vi "Body.vi"() -> ()   [LabVIEW 2011]
uses:
  <vilib>/Utility/miscctls.llb/LVPointTypeDef.ctl
  Globals/Global VI.vi
panel:
  out "Access Levels":i32[](array[numeric])
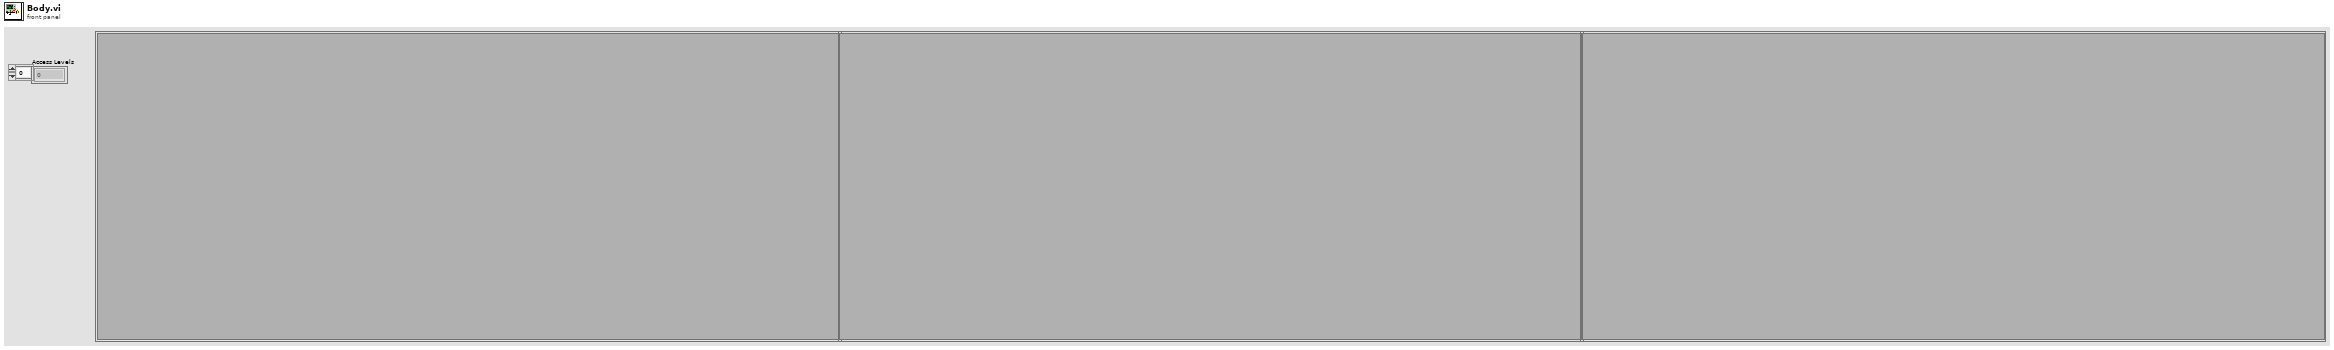
[diagram p1: front panel]
types:
  T1 = typedef "LVPointTypeDef.ctl" = cluster{"Horizontal":i16, "Vertical":i16}
  T2 = enum32{"Bad", "Idle", "Run top level", "Running"}
  T3 = enum8{"Enabled", "Disabled", "Disabled and Grayed Out"}
  T4 = enum16{"Always On", "Always Off", "Off While Running"}
  T5 = typedef "LVAllMonitorsDisplayTypeDef.ctl" = cluster{"Bounds":cluster{"Left":i16, "Top":i16, "Right":i16, "Bottom":i16}, "Depth":i16}[]
  T6 = typedef "LVRectTypeDef.ctl" = cluster{"left":i16, "top":i16, "right":i16, "bottom":i16}
  T7 = cluster{"Bounds":cluster{"Left":i16, "Top":i16, "Right":i16, "Bottom":i16}, "Depth":i16}
  T8 = typedef "LVBoundsTypeDef.ctl" = cluster{"Width":u32, "Height":u32}
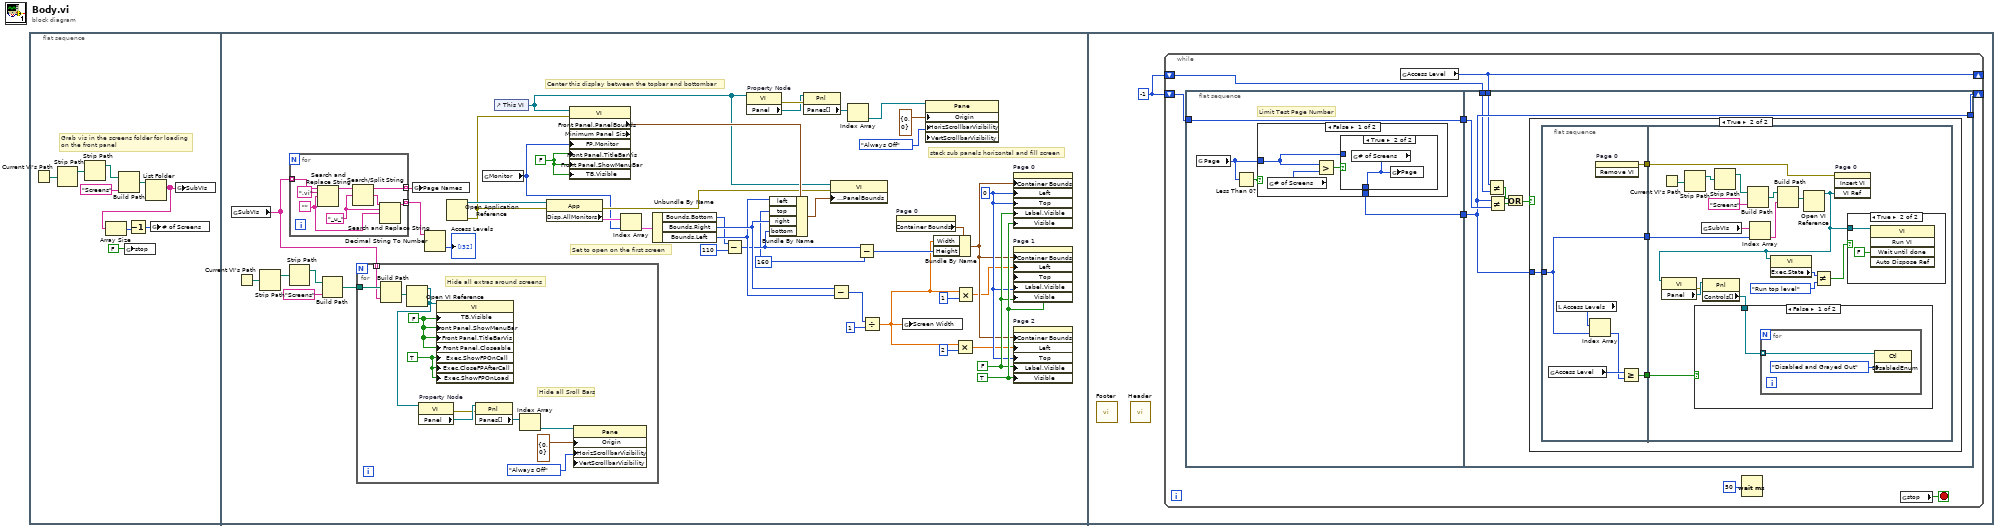
[diagram p0: block diagram]
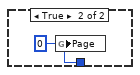
[diagram p3: hidden frame]
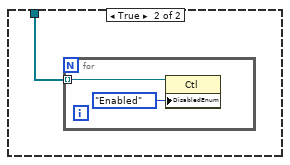
[diagram p6: hidden frame]
diagram:
  n1 = flat-sequence {
    frame #0 {
      # "Grab vis in the screens folder for loading\non the front panel"
      n2 = Current VI's Path() -> (path=w8:path)
      n3 = Strip Path(path=w8) -> (stripped path=w6:path)  [unwired: 1 out]
      n4 = Strip Path(path=w6) -> (stripped path=w5:path)  [unwired: 1 out]
      n5 = Build Path(base path=w5, name or relative path="Screens") -> (appended path=w7:path)
      n6 = global write "Global VI.vi" "stop"(FALSE ("stop")) -> ()
      n7 = List Folder(path=w7) -> (filenames=w2:string[])  [unwired: 3 in, 3 out]
      n8 = Array Size(array=w2) -> (size(s)=w3:i32)
      n9 = Decrement(x=w3) -> (x-1=w4:i32)
      n10 = global write "Global VI.vi" "# of Screens"(w4) -> ()
      n11 = global write "Global VI.vi" "SubVIs"(w2) -> ()
    }
    frame #1 {
      w13 = T4."Always Off" ("Horizontal Scrollbar Visibility")
      w15 = FALSE ("Front Panel Window:Title Bar Visible")
      w46 = TRUE ("Label.Visible")
      w45 = FALSE ("Label.Visible")
      w44 = 0 ("Position:Left")
      w36 = i16 160 ("top")
      # "Set to open on the first screen"
      # "stack sub panels horizontal and fill screen"
      # "Center this display between the topbar and bottombar"
      n12 = global read "Global VI.vi" "SubVIs"() -> (w21:string[])
      n13 = Current VI's Path() -> (path=w51:path)
      n14 = Strip Path(path=w51) -> (stripped path=w18:path)  [unwired: 1 out]
      n15 = for {
        tunnel: w21 -> [w73] mode=indexing
        tunnel: [w70] -> w12 mode=indexing
        tunnel: [w66] -> w11 mode=indexing
        w68 = "_u_" ("search string/char (-)")
        w67 = ""
        n16 = Search and Replace String(input string=w73, search string=".vi", replace string=w67) -> (result string=w71:string)  [unwired: 5 in, 3 out]
        n17 = Search/Split String(string=w71, search string/char (-)=w68) -> (substring before match=w70:string, match + rest of string=w69:string)  [unwired: 1 in, 1 out]
        n18 = Search and Replace String(input string=w69, search string=w68, replace string=w67) -> (result string=w66:string)  [unwired: 5 in, 3 out]
      }
      n19 = Strip Path(path=w18) -> (stripped path=w17:path)  [unwired: 1 out]
      n20 = Build Path(base path=w17, name or relative path="Screens") -> (appended path=w53:path)
      n21 = for {
        tunnel: w53 -> [w64]
        tunnel: w21 -> [w63] mode=indexing
        w60 = T4."Always Off" ("Horizontal Scrollbar Visibility")
        w61 = TRUE ("Execution:Show Front Panel On Call")
        w62 = FALSE ("Tool Bar:Visible")
        # "Hide all extras around screens"
        # "Hide all Sroll Bars"
        n22 = Build Path(base path=w64, name or relative path=w63) -> (appended path=w65:path)
        n23 = Open VI Reference(vi path=w65) -> (vi reference=w54:refnum<vi>)  [unwired: 5 in, 1 out]
        n24 = property on="Property Node" class="VI"(reference=w54) -> (error out=w57:errorcluster, "Panel"=w58:refnum<vi>)  [unwired: 1 in, 1 out]
        n25 = property class="VI"(reference=w54, "TB.Visible"=w62, "Front Panel.ShowMenuBar"=w62, "Front Panel.TitleBarVis"=w62, "Front Panel.Closeable"=w62, "Exec.ShowFPOnCall"=w61, "Exec.CloseFPAfterCall"=w61, "Exec.ShowFPOnLoad"=w61) -> ()  [unwired: 1 in, 2 out]
        n26 = property class="Pnl"(reference=w58, error in=w57) -> ("Panes[]"=w59:refnum<vi>[])  [unwired: 2 out]
        n27 = Index Array "Index Array"(array=w59) -> (element=w55:refnum<vi>)  [unwired: 1 in]
        n28 = property class="Pane"(reference=w55, "Origin"=T1 {"Horizontal"=0, "Vertical"=0}, "HorizScrollbarVisibility"=w60, "VertScrollbarVisibility"=w60) -> ()  [unwired: 1 in, 2 out]
      }
      n29 = global write "Global VI.vi" "Page Names"(w12) -> ()
      n30 = Decimal String To Number(string=w11) -> (number=→"Access Levels":i32[])  [unwired: 2 in, 1 out]
      n31 = Open Application Reference() -> (0:w27:errorcluster, 3:w33:refnum<vi>)  [unwired: 4 in]
      n32 = global read "Global VI.vi" "Monitor"() -> (w20:u16)
      n33 = control-ref of="This VI"() -> (w16:refnum<vi>)
      n34 = property class="App"(reference=w33, error in=w27) -> (error out=w24:errorcluster, "Disp.AllMonitors"=w23:T5)  [unwired: 1 out]
      n35 = property class="VI" props=["Front Panel.PanelBounds", "Minimum Panel Size", "FP.Monitor", "Front Panel.TitleBarVis", "Front Panel.ShowMenuBar", "TB.Visible"](reference=w16, error in=w27, "FP.Monitor"=w20, "Front Panel.TitleBarVis"=w15, "Front Panel.ShowMenuBar"=w15, "TB.Visible"=w15) -> ("Front Panel.PanelBounds"=w26:T6)  [unwired: 3 out]
      n36 = Index Array(array=w23, index=w20) -> (element=w22:T7)
      n37 = Unbundle By Name(w22) -> ("Bounds.Bottom"=w28:i16, "Bounds.Right"=w48:i16, "Bounds.Left"=w47:i16)
      n38 = Subtract(x=w28, y=i16 110) -> (x-y=w37:i16)
      n39 = property on="Property Node" class="VI"(reference=w16) -> (error out=w31:errorcluster, "Panel"=w30:refnum<vi>)  [unwired: 1 in, 1 out]
      n40 = Bundle By Name(cluster=w26, "left"=w47, "top"=w36, "right"=w48, "bottom"=w37) -> (w25:T6)
      n41 = property class="Pnl"(reference=w30, error in=w31) -> ("Panes[]"=w14:refnum<vi>[])  [unwired: 2 out]
      n42 = property class="VI"(reference=w16, error in=w24, "Front Panel.PanelBounds"=w25) -> ()  [unwired: 2 out]
      n43 = Subtract(x=w48, y=w47) -> (x-y=w49:i16)
      n44 = Index Array "Index Array"(array=w14) -> (element=w34:refnum<vi>)  [unwired: 1 in]
      n45 = Subtract(x=w37, y=w36) -> (x-y=w38:i16)
      n46 = Divide(x=w49, y=i16 1) -> (x/y=w19:dbl)
      n47 = property on="Page 0" class="SubPnl"() -> ("Container Bounds"=w35:T8)  [unwired: 2 in, 2 out]
      n48 = global write "Global VI.vi" "Screen Width"(w19) -> ()
      n49 = property class="Pane"(reference=w34, "Origin"=T1 {"Horizontal"=0, "Vertical"=0}, "HorizScrollbarVisibility"=w13, "VertScrollbarVisibility"=w13) -> ()  [unwired: 1 in, 2 out]
      n50 = Bundle By Name(cluster=w35, "Width"=w19, "Height"=w38) -> (w41:T8)
      n51 = Multiply(x=w19, y=i16 2) -> (x*y=w43:dbl)
      n52 = Multiply(x=w19, y=i16 1) -> (x*y=w40:dbl)
      n53 = property on="Page 0" class="SubPnl"("Container Bounds"=w41, "Left"=w44, "Top"=w44, "Label.Visible"=w45, "Visible"=w46) -> ()  [unwired: 2 in, 2 out]
      n54 = property on="Page 1" class="SubPnl"("Container Bounds"=w41, "Left"=w40, "Top"=w44, "Label.Visible"=w45, "Visible"=w46) -> ()  [unwired: 2 in, 2 out]
      n55 = property on="Page 2" class="SubPnl"("Container Bounds"=w41, "Left"=w43, "Top"=w44, "Label.Visible"=w45, "Visible"=w46) -> ()  [unwired: 2 in, 2 out]
    }
    frame #2 {
      w74 = i16 -1 ("Page")
      n56 = call "Footer.vi"() -> ()  [unwired: 12 in]
      n57 = call "Header.vi"() -> ()  [unwired: 12 in]
      n58 = while {
        shift-right: [w79] -> _
        shift-left: w74 -> [w80]
        shift-right: [w77] -> _
        shift-left: w74 -> [w76]
        stop <- w82 stop-if-true
        n59 = flat-sequence {
          tunnel: [w85] -> w81
          tunnel: w80 -> [w85]
          tunnel: [w83] -> w78
          tunnel: w81 -> [w100]
          tunnel: [w99] -> w79
          tunnel: w78 -> [w99]
          tunnel: w77 -> [w98]
          tunnel: w76 -> [w97]
          frame #0 {
            # "Limit Test Page Number"
            n60 = global read "Global VI.vi" "Page"() -> (w84:i16)
            n61 = Less Than 0?(x=w84) -> (x < 0?=w86:bool)
            n62 = case shown="False" w86 {
              tunnel: w84 -> [w87 _]
              tunnel: [w88 w93] -> w83
              frame False {
                n63 = global read "Global VI.vi" "# of Screens"() -> (w89:i16)
                n64 = Greater?(x=w87, y=w89) -> (0:w90:bool)
                n65 = case shown="True" w90 {
                  tunnel: [w91 w92] -> w88
                  tunnel: w87 -> [w91 _]
                  frame False {
                  }
                  frame True {
                    n66 = global read "Global VI.vi" "# of Screens"() -> (w92:i16)
                    n67 = global write "Global VI.vi" "Page"(w92) -> ()
                  }
                }
              }
              frame True {
                w93 = i16 0 ("Page")
                n68 = global write "Global VI.vi" "Page"(w93) -> ()
              }
            }
          }
          frame #1 {
            n69 = Not Equal?(x=w98, y=w97) -> (x != y?=w94:bool)
            n70 = Not Equal?(x=w99, y=w100) -> (x != y?=w95:bool)
            n71 = Or(x=w94, y=w95) -> (x .or. y?=w96:bool)
            n72 = case shown="True" w96 {
              tunnel: w99 -> [_ w103]
              frame False {
              }
              frame True {
                n73 = flat-sequence {
                  tunnel: [w110] -> w104
                  tunnel: w103 -> [w106]
                  tunnel: [w106] -> w102
                  tunnel: [w108] -> w101
                  tunnel: w104 -> [w120]
                  tunnel: w102 -> [w119]
                  tunnel: w101 -> [w115]
                  frame #0 {
                    n74 = global read "Global VI.vi" "Access Level"() -> (w109:u16)
                    n75 = local read "Access Levels"() -> (w107:i32[])
                    n76 = Index Array(array=w107, index=w106) -> (element=w105:i32)
                    n77 = invoke on="Page 0" class="SubPnl" method="Remove VI"() -> (error out=w110:errorcluster)  [unwired: 3 in, 2 out]
                    n78 = Greater Or Equal?(x=w109, y=w105) -> (x >= y?=w108:bool)
                  }
                  frame #1 {
                    n79 = Current VI's Path() -> (path=w127:path)
                    n80 = Strip Path(path=w127) -> (stripped path=w126:path)  [unwired: 1 out]
                    n81 = global read "Global VI.vi" "SubVIs"() -> (w122:string[])
                    n82 = Strip Path(path=w126) -> (stripped path=w125:path)  [unwired: 1 out]
                    n83 = Build Path(base path=w125, name or relative path="Screens") -> (appended path=w123:path)
                    n84 = Index Array(array=w122, index=w119) -> (element=w121:string)
                    n85 = Build Path(base path=w123, name or relative path=w121) -> (appended path=w124:path)
                    n86 = Open VI Reference(vi path=w124) -> (vi reference=w114:refnum<vi>)  [unwired: 5 in, 1 out]
                    n87 = property class="VI"(reference=w114) -> (error out=w117:errorcluster, "Panel"=w118:refnum<vi>)  [unwired: 1 in, 1 out]
                    n88 = property class="Pnl"(reference=w118, error in=w117) -> ("Controls[]"=w116:refnum<vi>[])  [unwired: 2 out]
                    n89 = case shown="False" w115 {
                      tunnel: w116 -> [w131 w134]
                      frame False {
                        n90 = for {
                          tunnel: w131 -> [w133] mode=indexing
                          n91 = property class="Ctl"(reference=w133, "DisabledEnum"=T3."Disabled and Grayed Out" ("Disabled")) -> ()  [unwired: 1 in, 2 out]
                        }
                      }
                      frame True {
                        n92 = for {
                          tunnel: w134 -> [w136] mode=indexing
                          n93 = property class="Ctl"(reference=w136, "DisabledEnum"=T3."Enabled" ("Disabled")) -> ()  [unwired: 1 in, 2 out]
                        }
                      }
                    }
                    n94 = property class="VI"(reference=w114) -> ("Exec.State"=w112:T2)  [unwired: 1 in, 2 out]
                    n95 = Not Equal?(x=w112, y=T2."Run top level" ("Execution:State")) -> (x != y?=w111:bool)
                    n96 = invoke on="Page 0" class="SubPnl" method="Insert VI"(error in=w120, "VI Ref"=w114) -> ()  [unwired: 2 in, 4 out]
                    n97 = case shown="True" w111 {
                      tunnel: w114 -> [_ w130]
                      frame False {
                      }
                      frame True {
                        n98 = invoke class="VI" method="Run VI"(reference=w130, "Wait until done"=FALSE ("Wait Until Done")) -> ()  [unwired: 3 in, 5 out]
                      }
                    }
                  }
                }
              }
            }
          }
        }
        n99 = global read "Global VI.vi" "Access Level"() -> (w77:u16)
        n100 = Wait (ms)(milliseconds to wait=u32 50) -> ()  [unwired: 1 out]
        n101 = global read "Global VI.vi" "stop"() -> (w82:bool)
      }
    }
  }
